vi "Hook Controller.vi"(8 "error in":errorcluster) -> ()   [LabVIEW 2019]
doc: "This VI executes continuously carrying out the current operation and responding to updates or new operations. It will often contain the timing or control code that is difficult to place directly in TeleOp. This VI generally opens all sensors and motors and isolates the rest of the robot code from knowing how the operations are carried out."
uses:
  <vilib>/Rock Robotics/WPI/Framework/Completion Status.ctl
  Hook Setpoints.ctl
  Hook Operations.ctl
  <vilib>/Rock Robotics/WPI/ThirdParty/Phoenix-LabVIEW/Motor Controller/Controls/CTRE_Phoenix_MotorControl_ControlMode.ctl
  <vilib>/Rock Robotics/Network Tables/NT Write Boolean.vi
panel:
  in  "Interactive Values":T1
  in  "Buttons":cluster{"Execute Cmd":bool, "Abort Cmd":bool}
  out "Command Timing":cluster{"Start Time (ms)":u32, "Iterations":i32}
  out "Status":T3
  # "Tip: It may be helpful to observe inputs and sensor values.\nYou may also want to display tuning or debugging controls."
  # "Interactive Command: You may fill in the settings for a command\nand schedule it with the Execute button. You can observe and abort\nany command while fine tuning the code for the controller."
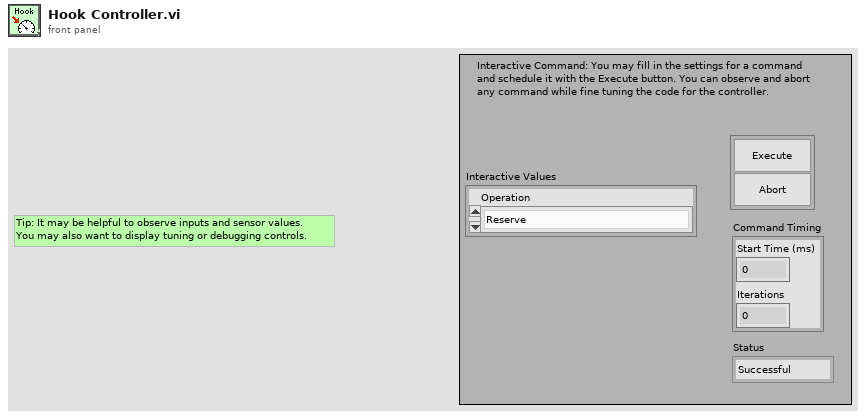
[diagram p1: front panel]
types:
  T1 = typedef "Hook Setpoints.ctl" = cluster{"Operation":T2}
  T2 = typedef "Hook Operations.ctl" = enum16{"Reserve", "Read Current", "Immediate", "Raise", "Lower", "Stop"}
  T3 = typedef "Completion Status.ctl" = enum16{"Successful", "Aborted", "Incomplete"}
  T4 = typedef "WPI_MotorControlDeviceRef.ctl" = cluster{"DeviceStatus":errorcluster, "Type":T5, "PWM":cluster{"PWM Channel":T6, "DeadBand":T7}, "CAN":cluster{"Device Number":u8, "SetOutput VI Ref":variant, "GetOutput VI Ref":variant, "Enable VI Ref":variant, "Disable VI Ref":variant, "Data":variant}, "Invert":bool, "DIO PWM":cluster{"PWM \"Enable\" Channel":T6, "DIOChannel":T8, "PWM Rate":dbl}}
  T5 = typedef "WPI_MotorControlType.ctl" = enum16{"PWM", "CAN", "DIO PWM"}
  T6 = typedef "FPGA_DIOPWMChannel.ctl" = enum8{"PWM 0", "PWM 1", "PWM 2", "PWM 3", "PWM 4", "PWM 5", "PWM 6", "PWM 7", "PWM 8", "PWM 9", "PWM MXP 0", "PWM MXP 1", "PWM MXP 2", "PWM MXP 3", "PWM MXP 4", "PWM MXP 5", "PWM MXP 6", "PWM MXP 7", "PWM MXP 8", "PWM MXP 9", "Invalid"}
  T7 = typedef "WPI_PWMDeadband.ctl" = cluster{"Name":string, "maxPositivePwm":i32, "minPositivePwm":i32, "centerPwm":i32, "maxNegativePwm":i32, "minNegativePwm":i32, "angularRange":u16}
  T8 = typedef "FPGA_DIOChannel.ctl" = enum8{"DIO 0", "DIO 1", "DIO 2", "DIO 3", "DIO 4", "DIO 5", "DIO 6", "DIO 7", "DIO 8", "DIO 9", "DIO MXP 0", "DIO MXP 1", "DIO MXP 2", "DIO MXP 3", "DIO MXP 4", "DIO MXP 5", "DIO MXP 6", "DIO MXP 7", "DIO MXP 8", "DIO MXP 9", "DIO MXP 10", "DIO MXP 11", "DIO MXP 12", "DIO MXP 13", "DIO MXP 14", "DIO MXP 15", "SPI Port CS1", "SPI Port CS2", "SPI Port CS3", "SPI Port MISO", "SPI Port MOSI", "Invalid"}
  T9 = typedef "Command Status Info.ctl" = cluster{"Name":string, "Status":T3, "notifier out":T10}
  T10 = typedef "Completion Notifier.ctl" = refnum<notifier>
  T11 = cluster{"Current Command":T1, "Command Timing":cluster{"Start Time (ms)":u32, "Iterations":i32}, "Command Arguments":cluster{"Command Info":T9, "Description":string, "Default Command":T1, "queue out":refnum<queue>, "Subsystem Name":string}}
  T12 = typedef "CTRE_Phoenix_MotorControl_ControlMode.ctl" = u16
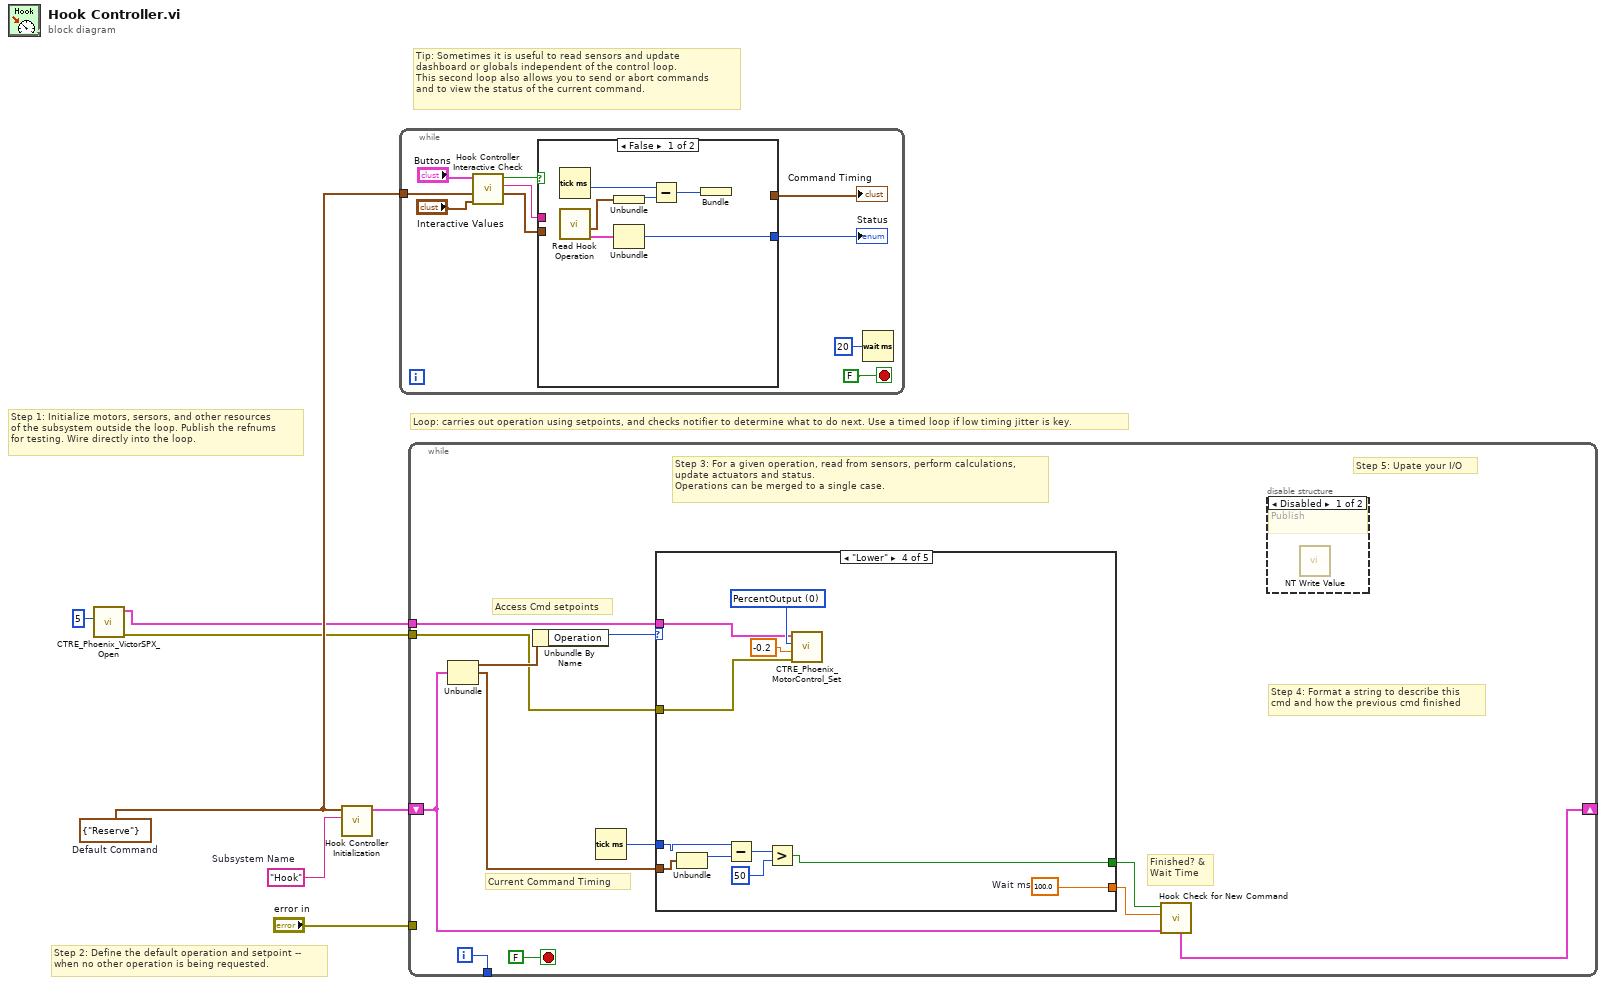
[diagram p0: block diagram]
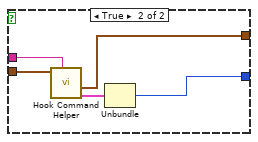
[diagram p2: hidden frame]
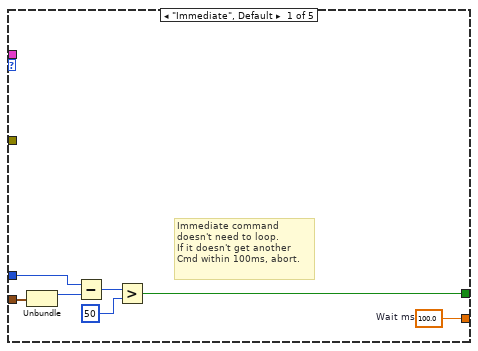
[diagram p4: hidden frame]
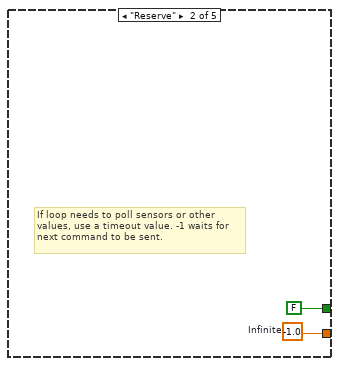
[diagram p5: hidden frame]
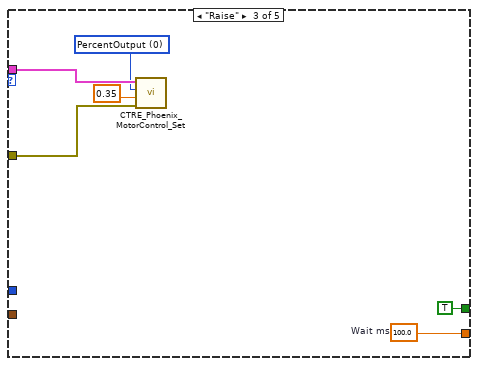
[diagram p6: hidden frame]
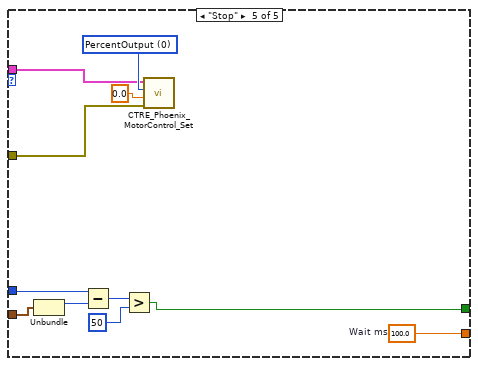
[diagram p7: hidden frame]
diagram:
  w4 = T1 {"Operation"=enum."Reserve"}  # Default Command
  w5 = "Hook"  # Subsystem Name
  # "Tip: Sometimes it is useful to read sensors and update\ndashboard or globals independent of the control loop.\nThis second loop also allows you to send or abort commands\nand to view the status of the current command."
  # "Step 2: Define the default operation and setpoint --\nwhen no other operation is being requested."
  # "Step 1: Initialize motors, sersors, and other resources\nof the subsystem outside the loop. Publish the refnums\nfor testing. Wire directly into the loop."
  # "Loop: carries out operation using setpoints, and checks notifier to determine what to do next. Use a timed loop if low timing jitter is key."
  n1 = call <vilib>:"CTRE_Phoenix_VictorSPX_Open.vi"("Device Number"=u8 5) -> ("error out"=w1:errorcluster, "CAN Talon SRX Ref"=w2:T4)  [unwired: 9 in]
  n2 = call "Hook Controller Initialization.vi"("Subsystem Name"=w5, "Default Command"=w4) -> ("Current Command"=w6:T11)  [unwired: 9 in]
  n3 = while {
    tunnel: w4 -> [w14]
    stop <- FALSE stop-if-true
    n4 = call "Hook Controller Interactive Check.vi"("Interactive Command in"="Interactive Values", "Default Command"=w14, "Buttons"="Buttons") -> ("Interactive Command out"=w11:T1, "Trace String"=w12:string, "Schedule"=w13:bool)  [unwired: 6 in]
    n5 = case shown="False" w13 {
      tunnel: [w23 w28] -> w10
      tunnel: w11 -> [_ w26]
      tunnel: [_ w24] -> w9
      tunnel: w12 -> [_ w27]
      frame False {
        n6 = Tick Count (ms)() -> (millisecond timer value=w20:u32)
        n7 = call "Read Hook Operation.vi"() -> ("Command Info"=w18:T9, "SubSystem Data"=w19:T1)  [unwired: 9 in, 1 out]
        n8 = Unbundle(w19) -> ("Operation"=w22:T2)
        n9 = Unbundle(w18) -> ("Status"=w23:T3)  [unwired: 2 out]
        n10 = Subtract(x=w20, y=w22) -> (x-y=w21:u32)
        n11 = Bundle(w21) -> ()  [unwired: 1 in, 1 out]
      }
      frame True {
        n12 = call "Hook Command Helper.vi"("Description"=w27, "SubSystem Data"=w26) -> ("Command Info Out"=w25:T9, "Command Timing"=w24:cluster{"Start Time (ms)":u32, "Iterations":i32})  [unwired: 7 in, 1 out]
        n13 = Unbundle(w25) -> ("Status"=w28:T3)  [unwired: 2 out]
      }
    }
    "Status" <- w10
    "Command Timing" <- w9
    n14 = Wait (ms)(milliseconds to wait=u32 20) -> ()  [unwired: 1 out]
  }
  n15 = while {
    shift-right: [w34] -> _
    shift-left: w6 -> [w31]
    tunnel: [w39] -> _
    tunnel: "error in" -> [_]
    tunnel: w2 -> [w30]
    tunnel: w1 -> [w29]
    i -> [w39]
    stop <- FALSE stop-if-true
    # "Step 5: Upate your I/O"
    # "Step 4: Format a string to describe this\ncmd and how the previous cmd finished"
    # "Current Command Timing"
    # "Access Cmd setpoints"
    # "Finished? &\nWait Time"
    # "Step 3: For a given operation, read from sensors, perform calculations,\nupdate actuators and status.\nOperations can be merged to a single case."
    n16 = Unbundle(w31) -> ("Current Command"=w38:T1, "Command Timing"=w35:cluster{"Start Time (ms)":u32, "Iterations":i32})  [unwired: 1 out]
    n17 = Unbundle By Name(w38) -> ("Operation"=w37:T2)
    n18 = Tick Count (ms)() -> (millisecond timer value=w36:u32)
    n19 = case shown="\"Lower\"" w37 {
      tunnel: [w47 w49 w51 w56 w67] -> w32
      tunnel: [w41 FALSE ("ignore previous (F)") TRUE ("ignore previous (F)") w57 w68] -> w33
      tunnel: w35 -> [w43 _ _ w59 w70]
      tunnel: w36 -> [w42 _ _ w58 w69]
      tunnel: w30 -> [_ _ w55 w64 w74]
      tunnel: w29 -> [_ _ w54 w63 w75]
      frame "Immediate", Default {
        w47 = 100.0  # Wait ms
        # "Immediate command\ndoesn't need to loop.\nIf it doesn't get another\nCmd within 100ms, abort."
        n20 = Unbundle(w43) -> ("Start Time (ms)"=w46:u32)  [unwired: 1 out]
        n21 = Subtract(x=w42, y=w46) -> (x-y=w45:u32)
        n22 = Greater?(x=w45, y=u8 50 ("Left Motor")) -> (0:w41:bool)
      }
      frame "Reserve" {
        w49 = -1.0  # Infinite
        # "If loop needs to poll sensors or other\nvalues, use a timeout value. -1 waits for\nnext command to be sent."
      }
      frame "Raise" {
        w51 = 100.0  # Wait ms
        w53 = T12 0 items=["PercentOutput"=0, "Position"=1, "Velocity"=2, "Current"=3, "Follower"=5, "MotionProfile"=6, "MotionMagic"=7, "MotionProfileArc"=10, "Disabled"=15] ("Control Mode")
        n23 = call <vilib>:"CTRE_Phoenix_MotorControl_Set.vi"("error in (no error)"=w54, "Output"=0.35, "Control Mode"=w53, "PhoenixMotorControlDevRef"=w55) -> ()  [unwired: 6 in, 2 out]
      }
      frame "Lower" {
        w56 = 100.0  # Wait ms
        w66 = T12 0 items=["PercentOutput"=0, "Position"=1, "Velocity"=2, "Current"=3, "Follower"=5, "MotionProfile"=6, "MotionMagic"=7, "MotionProfileArc"=10, "Disabled"=15] ("Control Mode")
        n24 = Unbundle(w59) -> ("Start Time (ms)"=w60:u32)  [unwired: 1 out]
        n25 = Subtract(x=w58, y=w60) -> (x-y=w61:u32)
        n26 = Greater?(x=w61, y=u8 50 ("Left Motor")) -> (0:w57:bool)
        n27 = call <vilib>:"CTRE_Phoenix_MotorControl_Set.vi"("error in (no error)"=w63, "Output"=-0.2, "Control Mode"=w66, "PhoenixMotorControlDevRef"=w64) -> ()  [unwired: 6 in, 2 out]
      }
      frame "Stop" {
        w67 = 100.0  # Wait ms
        w77 = T12 0 items=["PercentOutput"=0, "Position"=1, "Velocity"=2, "Current"=3, "Follower"=5, "MotionProfile"=6, "MotionMagic"=7, "MotionProfileArc"=10, "Disabled"=15] ("Control Mode")
        n28 = Unbundle(w70) -> ("Start Time (ms)"=w71:u32)  [unwired: 1 out]
        n29 = Subtract(x=w69, y=w71) -> (x-y=w72:u32)
        n30 = Greater?(x=w72, y=u8 50 ("Left Motor")) -> (0:w68:bool)
        n31 = call <vilib>:"CTRE_Phoenix_MotorControl_Set.vi"("error in (no error)"=w75, "Output"=0.0, "Control Mode"=w77, "PhoenixMotorControlDevRef"=w74) -> ()  [unwired: 6 in, 2 out]
      }
    }
    n32 = call "Hook Check for New Command.vi"("Current Command"=w31, "Wait time (ms)"=w32, "Finished?"=w33) -> ("NextCommand"=w34:T11)  [unwired: 4 in, 4 out]
    n33 = disable-structure shown="Disabled" {
      frame Disabled {
        # "Publish"
        n34 = call-poly <vilib>:"NT Write Value.vi"() -> ()  [unwired: 11 in, 1 out]
      }
      frame Enabled {
      }
    }
  }
